vi "Initialize Python Global Variables.vi"(7 "Server Alias":string, 8 "Error In":errorcluster) -> (0 "Error Out":errorcluster)   [LabVIEW 2013, in "TS.lvlib"]
uses:
  TS.lvlib
  LabVIEW Example/Supporting Code/Script Running.ctl
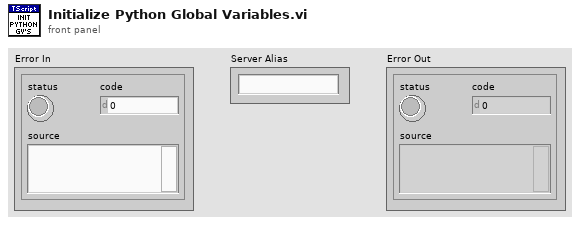
[diagram p1: front panel]
types:
  T1 = typedef "TS.lvlib/Script Running.ctl" = cluster{"Script ID":i64, "Script Running?":bool}
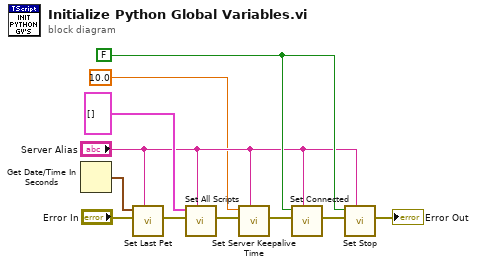
[diagram p0: block diagram]
diagram:
  w6 = FALSE
  n1 = Get Date/Time In Seconds() -> (seconds since 1Jan1904=w8:timestamp)
  n2 = call "Set Last Pet.vi"("Server Alias"="Server Alias", "Error In"="Error In", "Last Pet"=w8) -> ("Error Out"=w11:errorcluster)  [unwired: 8 in]
  n3 = call "Set All Scripts.vi"("Server Alias"="Server Alias", "Error In"=w11, "All Scripts"=T1[] []) -> ("Error Out"=w10:errorcluster)  [unwired: 8 in]
  n4 = call "Set Server Keepalive Time.vi"("Server Alias"="Server Alias", "Error In"=w10, "Server Keepalive Time"=10.0) -> ("Error Out"=w3:errorcluster)  [unwired: 8 in]
  n5 = call "Set Connected.vi"("Server Alias"="Server Alias", "Error In"=w3, "Connected"=w6) -> ("Error Out"=w9:errorcluster)  [unwired: 8 in]
  n6 = call "Set Stop.vi"("Server Alias"="Server Alias", "Error In"=w9, "Stop"=w6) -> ("Error Out"=→"Error Out":errorcluster)  [unwired: 8 in]
